vi "Configure RemIO Module Core.vi"(8 "error in (no error)":errorcluster, 9 "module slot index":u8=1, 10 "Slave Ref In":refnum<k21>, 11 "11152 in":refnum<class "11152.lvclass">) -> (0 "error out":errorcluster, 1 "negative confirmation":T1 {"additional error code" format="%.0x"; "error code" format="%.0x"}, 2 "Slave Ref Out":refnum<k21>, 3 "11152 out":refnum<class "11152.lvclass">, 5 "SDO abort code":u32 format="%.0x")   [LabVIEW 2017, in "Modules.lvlib" / "11152.lvclass"]
uses:
  11152.lvclass
  <vilib>/indcomecat/Remote IO/typedefs/negative confirmation.ctl
  11152.lvclass/11152.ctl
  f84f802e-5f49-4222-a062-bef69e82b192.vi
  RemIO Module/Get RemIO Library Path.vi
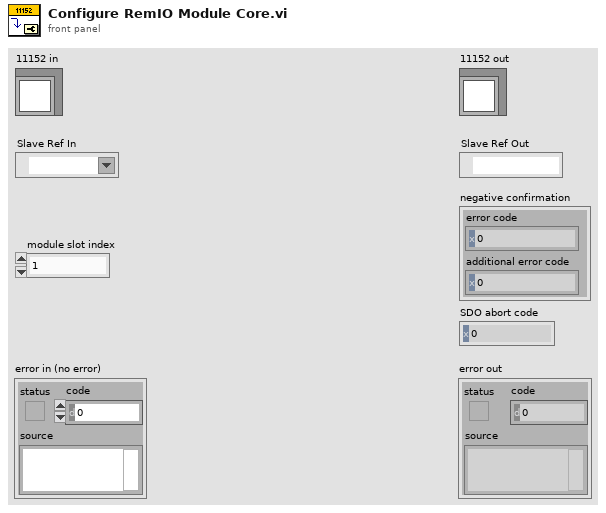
[diagram p1: front panel]
types:
  T1 = typedef "negative confirmation.ctl" = cluster{"error code":u16, "additional error code":u16}
  T2 = typedef "NI ECAT Remote IO.lvlib/input filter time REM-11152.ctl" = u8
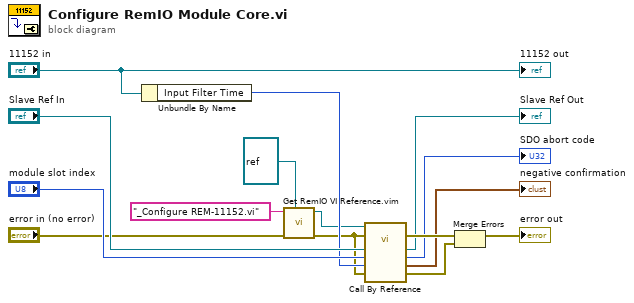
[diagram p0: block diagram]
diagram:
  n1 = Unbundle By Name("11152 in") -> ("Input Filter Time"=w6:T2)
  n2 = call "Get RemIO VI Reference.vim"("name or relative path"="_Configure REM-11152.vi", "error in (no error)"="error in (no error)", "type specifier VI Refnum (for type only)"=refnum<vi> refnum) -> ("vi reference"=w1:refnum<vi>, "error out"=w4:errorcluster)  [unwired: 6 in]
  n3 = call-by-ref "?"(reference=w1, error in=w4, 8:"error in (no error)"=w4, "input filter time"=w6, "module slot index"="module slot index", "slave reference in"="Slave Ref In") -> (error out=w13:errorcluster, 0:"error out"=w14:errorcluster, "negative confirmation"=→"negative confirmation":T1, "SDO abort code"=→"SDO abort code":u32, "slave reference out"=→"Slave Ref Out":refnum<k21>)  [unwired: 4 in, 1 out]
  n4 = Merge Errors(w13, w14) -> (→"error out":errorcluster)
  "11152 out" <- "11152 in"
